vi "girpcutil_RpcValue_Set.vi"(0 "girpcutil_params":T2, 1 "StringValue or Snippet":string, 2 "Int32Value or struct":i32, 3 "Int64Value":i64, 4 "DoubleValue":dbl, 5 "FloatValue":sgl, 6 "BoolValue":bool=TRUE, 7 "Fehler (Eingang, kein Fehler)":errorcluster, 10 "MemberName":string, 12 "param handle":i32, 14 "DataType":T1(ring)) -> (27 "Fehler (Ausgang)":errorcluster)   [LabVIEW 2016]
uses:
  girpcutil_params.ctl
panel:
  out "errMsg":u8[](array[numeric])
  out "errMsgLen":i32
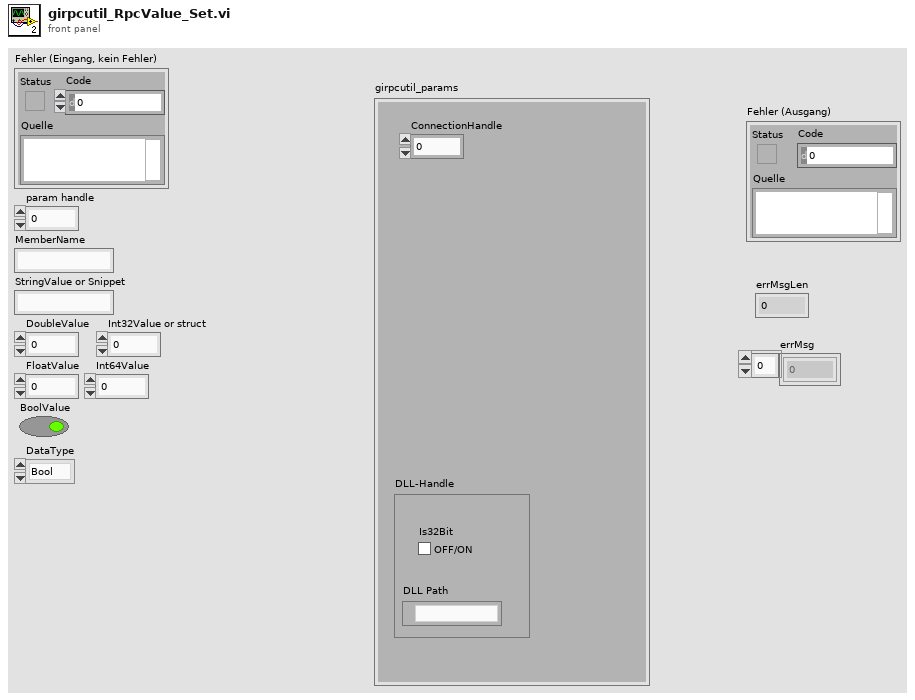
[diagram p1: front panel]
types:
  T1 = enum16{"Bool", "Snippet", "Struct", "Int64", "Int32", "Float", "Double", "String"}
  T2 = typedef "girpcutil_params.ctl" = cluster{"ConnectionHandle":i32, "DLL-Handle":cluster{"DLL Path":path, "Is32Bit":bool}}
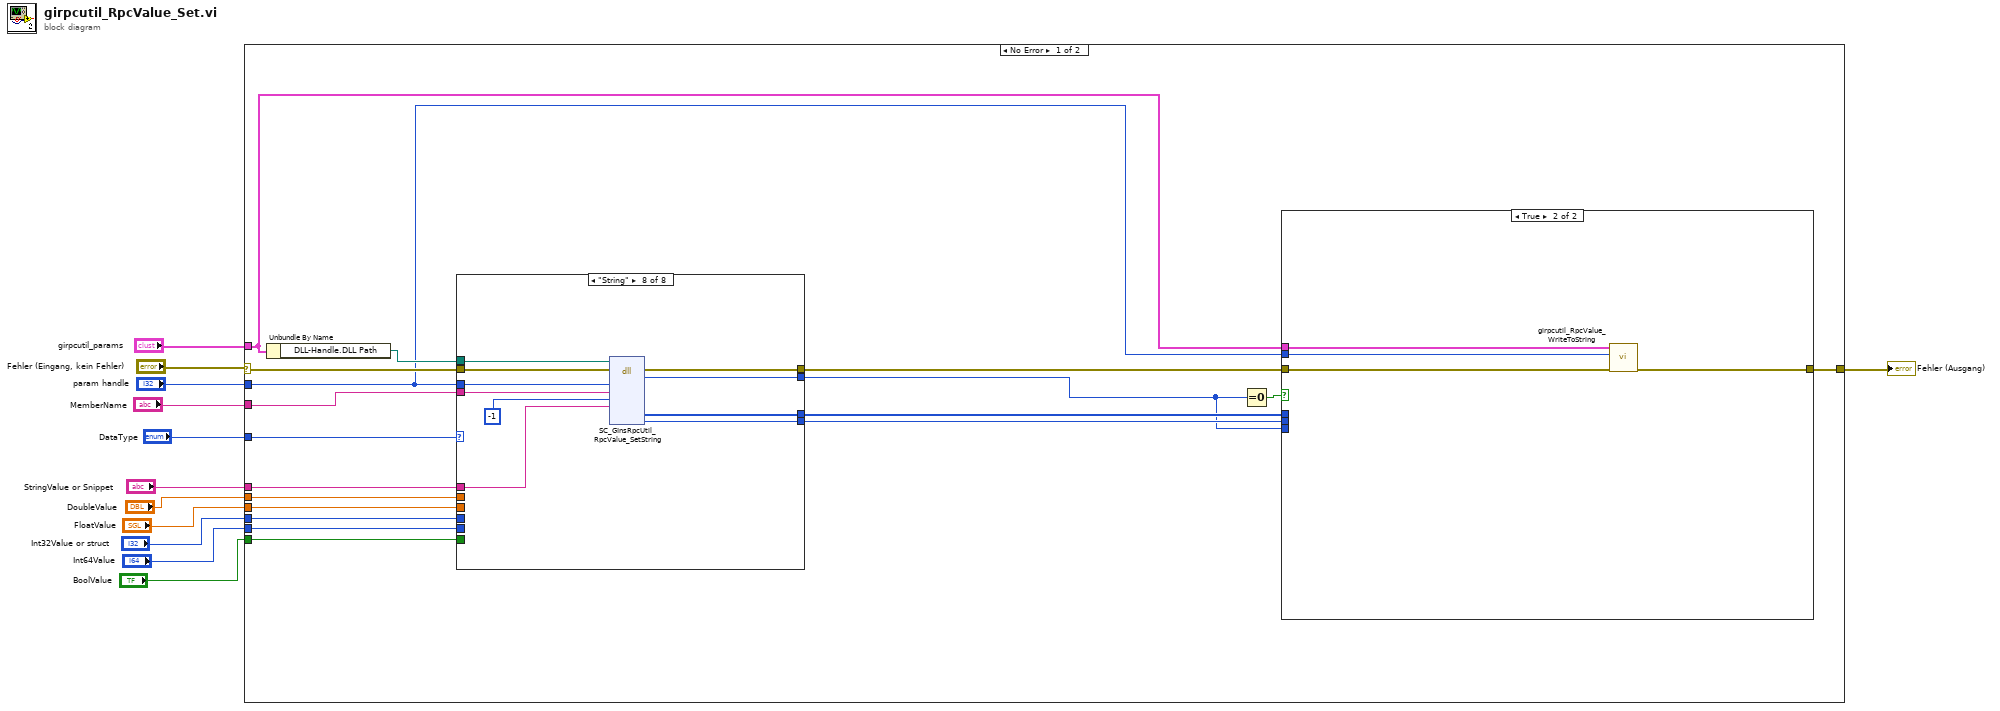
[diagram p0: block diagram]
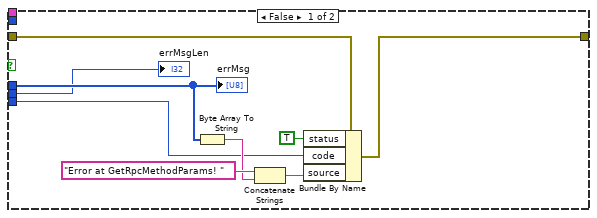
[diagram p2: hidden frame]
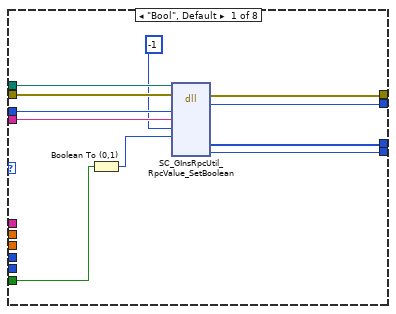
[diagram p3: hidden frame]
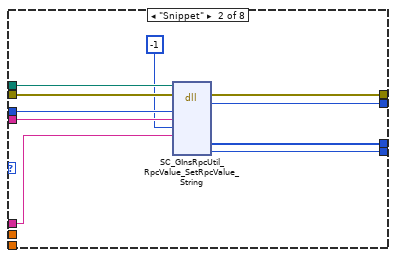
[diagram p4: hidden frame]
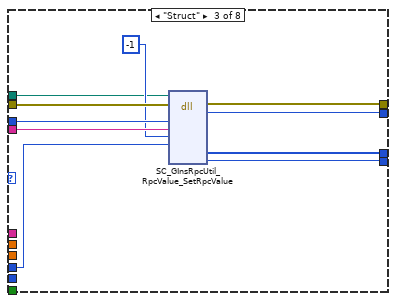
[diagram p5: hidden frame]
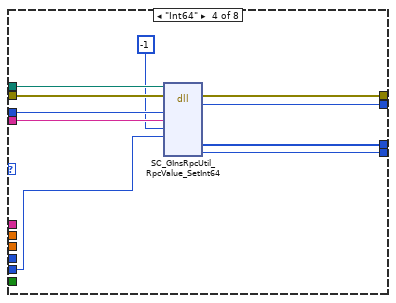
[diagram p6: hidden frame]
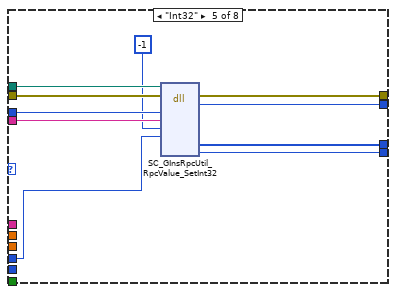
[diagram p7: hidden frame]
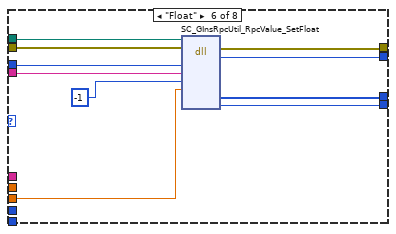
[diagram p8: hidden frame]
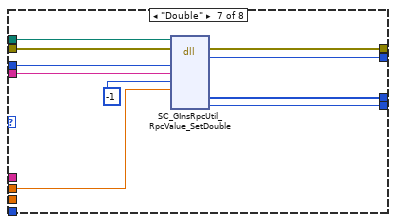
[diagram p9: hidden frame]
diagram:
  n1 = case shown="No Error" "Fehler (Eingang, kein Fehler)" {
    selector: "Fehler (Eingang, kein Fehler)" -> [w29 w125]
    tunnel: [w13 w125] -> w11
    tunnel: "DataType" -> [w30 _]
    tunnel: "girpcutil_params" -> [w22 _]
    tunnel: "param handle" -> [w23 _]
    tunnel: "MemberName" -> [w27 _]
    tunnel: "StringValue or Snippet" -> [w26 _]
    tunnel: "DoubleValue" -> [w18 _]
    tunnel: "FloatValue" -> [w17 _]
    tunnel: "Int32Value or struct" -> [w16 _]
    tunnel: "Int64Value" -> [w15 _]
    tunnel: "BoolValue" -> [w14 _]
    frame No Error {
      n2 = Unbundle By Name(w22) -> ("DLL-Handle.DLL Path"=w28:path)
      n3 = case shown="\"String\"" w30 {
        tunnel: w29 -> [w54 w64 w74 w84 w94 w104 w113 w124]
        tunnel: w28 -> [w52 w62 w65 w82 w92 w102 w114 w123]
        tunnel: w23 -> [w51 w61 w72 w81 w91 w101 w111 w122]
        tunnel: w27 -> [w50 w60 w71 w80 w90 w100 w110 w121]
        tunnel: w26 -> [_ w55 _ _ _ _ _ w119]
        tunnel: [w49 w59 w70 w79 w87 w96 w105 w118] -> w19
        tunnel: [w53 w63 w73 w83 w93 w103 w112 w117] -> w24
        tunnel: [w47 w57 w68 w77 w88 w97 w106 w116] -> w21
        tunnel: [w48 w58 w69 w78 w89 w98 w107 w115] -> w20
        tunnel: w18 -> [_ _ _ _ _ _ w108 _]
        tunnel: w17 -> [_ _ _ _ _ w95 _ _]
        tunnel: w16 -> [_ _ w66 _ w85 _ _ _]
        tunnel: w15 -> [_ _ _ w75 _ _ _ _]
        tunnel: w14 -> [w45 _ _ _ _ _ _ _]
        frame "Bool", Default {
          n4 = Boolean To (0,1)(Boolean=w45) -> (0, 1=w46:i16)
          n5 = dll-call lib="?" fn="SC_GInsRpcUtil_RpcValue_SetBoolean"(path in=w52, error in=w54, "dest"=w51, "member"=w50, "index"=-1, "value"=w46) -> (error out=w53:errorcluster, "Rückgabewert"=w49:i32, "errMsg"=w48:u8[], "errMsgLen"=w47:i32)  [unwired: 7 in, 1 out]
        }
        frame "Snippet" {
          n6 = dll-call lib="?" fn="SC_GInsRpcUtil_RpcValue_SetRpcValue_String"(path in=w62, error in=w64, "dest"=w61, "member"=w60, "index"=-1, "value"=w55) -> (error out=w63:errorcluster, "Rückgabewert"=w59:i32, "errMsg"=w58:u8[], "errMsgLen"=w57:i32)  [unwired: 7 in, 1 out]
        }
        frame "Struct" {
          n7 = dll-call lib="?" fn="SC_GInsRpcUtil_RpcValue_SetRpcValue"(path in=w65, error in=w74, "dest"=w72, "member"=w71, "index"=-1, "value"=w66) -> (error out=w73:errorcluster, "Rückgabewert"=w70:i32, "errMsg"=w69:u8[], "errMsgLen"=w68:i32)  [unwired: 7 in, 1 out]
        }
        frame "Int64" {
          n8 = dll-call lib="?" fn="SC_GInsRpcUtil_RpcValue_SetInt64"(path in=w82, error in=w84, "dest"=w81, "member"=w80, "index"=-1, "value"=w75) -> (error out=w83:errorcluster, "Rückgabewert"=w79:i32, "errMsg"=w78:u8[], "errMsgLen"=w77:i32)  [unwired: 7 in, 1 out]
        }
        frame "Int32" {
          n9 = dll-call lib="?" fn="SC_GInsRpcUtil_RpcValue_SetInt32"(path in=w92, error in=w94, "dest"=w91, "member"=w90, "index"=-1, "value"=w85) -> (error out=w93:errorcluster, "Rückgabewert"=w87:i32, "errMsg"=w89:u8[], "errMsgLen"=w88:i32)  [unwired: 7 in, 1 out]
        }
        frame "Float" {
          n10 = dll-call lib="?" fn="SC_GInsRpcUtil_RpcValue_SetFloat"(path in=w102, error in=w104, "dest"=w101, "member"=w100, "index"=-1, "value"=w95) -> (error out=w103:errorcluster, "Rückgabewert"=w96:i32, "errMsg"=w98:u8[], "errMsgLen"=w97:i32)  [unwired: 7 in, 1 out]
        }
        frame "Double" {
          n11 = dll-call lib="?" fn="SC_GInsRpcUtil_RpcValue_SetDouble"(path in=w114, error in=w113, "dest"=w111, "member"=w110, "index"=-1, "value"=w108) -> (error out=w112:errorcluster, "Rückgabewert"=w105:i32, "errMsg"=w107:u8[], "errMsgLen"=w106:i32)  [unwired: 7 in, 1 out]
        }
        frame "String" {
          n12 = dll-call lib="?" fn="SC_GInsRpcUtil_RpcValue_SetString"(path in=w123, error in=w124, "dest"=w122, "member"=w121, "index"=-1, "value"=w119) -> (error out=w117:errorcluster, "Rückgabewert"=w118:i32, "errMsg"=w115:u8[], "errMsgLen"=w116:i32)  [unwired: 7 in, 1 out]
        }
      }
      n13 = Equal To 0?(x=w19) -> (x = 0?=w25:bool)
      n14 = case shown="True" w25 {
        tunnel: w24 -> [w33 w43]
        tunnel: [w32 w42] -> w13
        tunnel: w20 -> [w37 _]
        tunnel: w21 -> [w34 _]
        tunnel: w19 -> [w31 _]
        tunnel: w23 -> [_ w41]
        tunnel: w22 -> [_ w40]
        frame False {
          n15 = Byte Array To String(unsigned byte array=w37) -> (string=w38:string)
          n16 = Concatenate Strings("Error at GetRpcMethodParams! " ("source"), w38) -> (w36:string)
          n17 = Bundle By Name(cluster=w33, "status"=TRUE, "code"=w31, "source"=w36) -> (w32:errorcluster)
          "errMsg" <- w37
          "errMsgLen" <- w34
        }
        frame True {
          n18 = call "girpcutil_RpcValue_WriteToString.vi"("Fehler (Eingang, kein Fehler)"=w43, "value"=w41, "girpcutil_params"=w40) -> ("Fehler (Ausgang)"=w42:errorcluster)  [unwired: 8 in]
        }
      }
    }
    frame Error {
    }
  }
  "Fehler (Ausgang)" <- w11
